vi "Step_2_Ans.vi"   [LabVIEW 2012]
types:
  T1 = typedef "BotSpeak_Control.ctl" = cluster{"Address":string, "Reply EOF":string, "Hardware":string, "Retries":i8, "Timeout":i32}
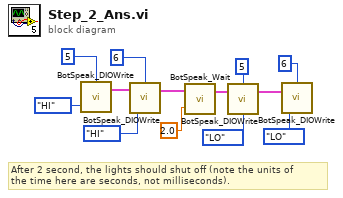
[diagram p0: block diagram]
diagram:
  # "After 2 second, the lights should shut off (note the units of\nthe time here are seconds, not milliseconds)."
  n1 = call <userlib>:"BotSpeak_DIOWrite.vi"("State"=enum32{"LO", "HI"}."HI", "DIO Line"=u32 5) -> ("Bot Settings"=w11:T1)  [unwired: 1 in, 1 out]
  n2 = call <userlib>:"BotSpeak_DIOWrite.vi"("State"=enum32{"LO", "HI"}."HI", "Bot Settings"=w11, "DIO Line"=u32 6) -> ("Bot Settings"=w8:T1)  [unwired: 1 out]
  n3 = call <userlib>:"BotSpeak_Wait.vi"("Wait (sec)"=2.0, "Bot Settings"=w8) -> ("Bot Settings"=w1:T1)  [unwired: 1 in]
  n4 = call <userlib>:"BotSpeak_DIOWrite.vi"("State"=enum32{"LO", "HI"}."LO", "Bot Settings"=w1, "DIO Line"=u32 5) -> ("Bot Settings"=w4:T1)  [unwired: 1 out]
  n5 = call <userlib>:"BotSpeak_DIOWrite.vi"("State"=enum32{"LO", "HI"}."LO", "Bot Settings"=w4, "DIO Line"=u32 6) -> ()  [unwired: 2 out]
